vi "File types.vi"(0 "file type 1":string, 1 "file type 2":string, 2 "file type 3":string, 3 "file type 4":string, 4 "file type 5":string, 5 "file type 6":string) -> (16 "Array":string[](array[string]))   [LabVIEW 2011]
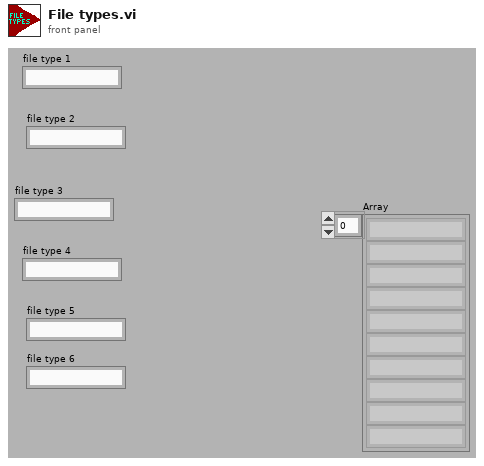
[diagram p1: front panel]
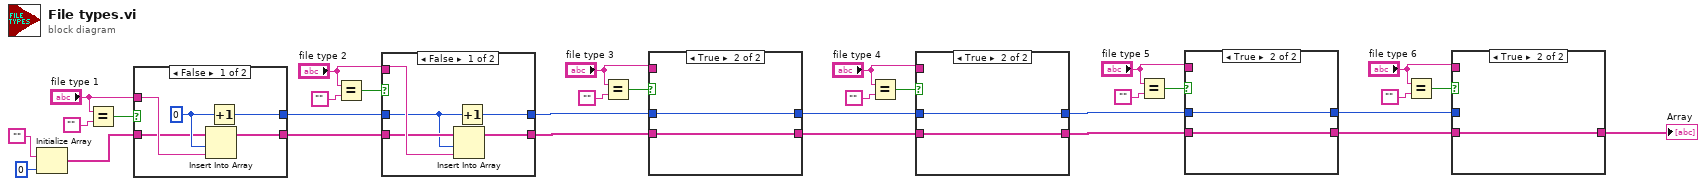
[diagram p0: block diagram]
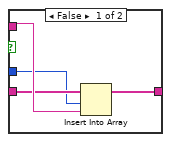
[diagram p2: hidden frame]
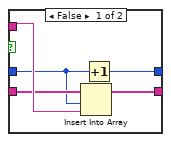
[diagram p3: hidden frame]
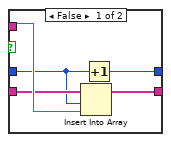
[diagram p4: hidden frame]
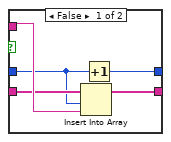
[diagram p5: hidden frame]
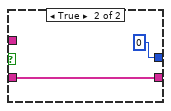
[diagram p7: hidden frame]
diagram:
  n1 = Initialize Array("", 0 ("dimension size")) -> (w27:string[])
  n2 = Equal?(x="file type 1", y="") -> (x = y?=w29:bool)
  n3 = case shown="False" w29 {
    tunnel: "file type 1" -> [w36 _]
    tunnel: [w35 0] -> w22
    tunnel: w27 -> [w34 w38]
    tunnel: [w33 w38] -> w23
    frame False {
      w37 = 0 ("index")
      n4 = Insert Into Array(array=w34, index=w37, new element=w36) -> (w33:string[])
      n5 = Increment(x=w37) -> (x+1=w35:i32)
    }
    frame True {
    }
  }
  n6 = Equal?(x="file type 2", y="") -> (x = y?=w25:bool)
  n7 = case shown="False" w25 {
    tunnel: "file type 2" -> [w44 _]
    tunnel: [w43 w46] -> w15
    tunnel: [w42 w45] -> w14
    tunnel: w23 -> [w41 w45]
    tunnel: w22 -> [w40 w46]
    frame False {
      n8 = Insert Into Array(array=w41, index=w40, new element=w44) -> (w42:string[])
      n9 = Increment(x=w40) -> (x+1=w43:i32)
    }
    frame True {
    }
  }
  n10 = Equal?(x="file type 3", y="") -> (x = y?=w20:bool)
  n11 = case shown="True" w20 {
    tunnel: "file type 3" -> [w51 _]
    tunnel: [w50 w53] -> w13
    tunnel: [w49 w52] -> w12
    tunnel: w14 -> [w48 w52]
    tunnel: w15 -> [w47 w53]
    frame False {
      n12 = Insert Into Array(array=w48, index=w47, new element=w51) -> (w49:string[])
      n13 = Increment(x=w47) -> (x+1=w50:i32)
    }
    frame True {
    }
  }
  n14 = Equal?(x="file type 4", y="") -> (x = y?=w17:bool)
  n15 = case shown="True" w17 {
    tunnel: "file type 4" -> [w58 _]
    tunnel: [w57 w60] -> w3
    tunnel: [w56 w59] -> w2
    tunnel: w12 -> [w55 w59]
    tunnel: w13 -> [w54 w60]
    frame False {
      n16 = Insert Into Array(array=w55, index=w54, new element=w58) -> (w56:string[])
      n17 = Increment(x=w54) -> (x+1=w57:i32)
    }
    frame True {
    }
  }
  n18 = Equal?(x="file type 5", y="") -> (x = y?=w5:bool)
  n19 = case shown="True" w5 {
    tunnel: "file type 5" -> [w65 _]
    tunnel: [w64 w67] -> w10
    tunnel: [w63 w66] -> w11
    tunnel: w2 -> [w62 w66]
    tunnel: w3 -> [w61 w67]
    frame False {
      n20 = Insert Into Array(array=w62, index=w61, new element=w65) -> (w63:string[])
      n21 = Increment(x=w61) -> (x+1=w64:i32)
    }
    frame True {
    }
  }
  n22 = Equal?(x="file type 6", y="") -> (x = y?=w8:bool)
  n23 = case shown="True" w8 {
    tunnel: "file type 6" -> [w71 _]
    tunnel: [w70 w72] -> w1
    tunnel: w11 -> [w69 w72]
    tunnel: w10 -> [w68 _]
    frame False {
      n24 = Insert Into Array(array=w69, index=w68, new element=w71) -> (w70:string[])
    }
    frame True {
    }
  }
  "Array" <- w1
